vi "Initialize Master.vi"(8 "error in":errorcluster, 11 "Serial Master in":refnum<class "Serial Master.lvclass">) -> (0 "error out":errorcluster, 3 "Serial Master out":refnum<class "Serial Master.lvclass">)   [LabVIEW 2013, in "Modbus Library - Advance.lvlib" / "Serial Master.lvclass"]
doc: "This provides an interface for the master to open a connection to the slave."
uses:
  Serial Master.lvclass
  Serial Master.lvclass/Serial Master.ctl
  Transmission Data Unit/Serial Interface/Serial Data Unit.lvclass
  Read VISA resource name.vi
  Read Serial Data Unit.vi
  Read Baud Rate.vi
  Read Parity.vi
  Read Flow Control.vi
  Serial Shared Components/Serial Shared Components.lvlib
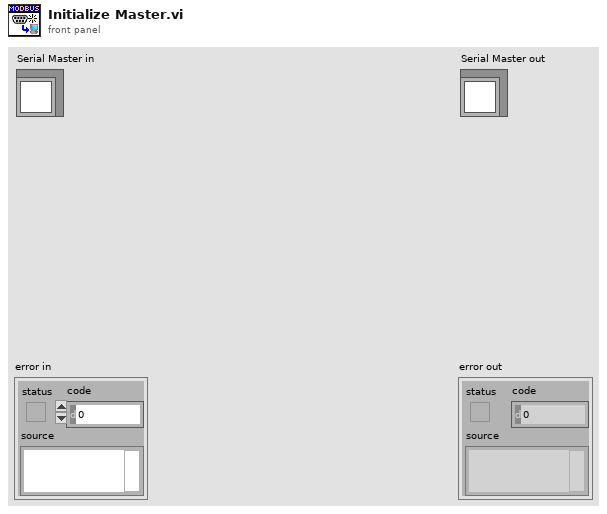
[diagram p1: front panel]
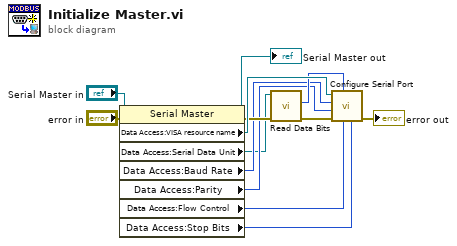
[diagram p0: block diagram]
diagram:
  n1 = property class="Serial Master"(reference="Serial Master in", error in="error in") -> (reference out=→"Serial Master out":refnum<class "Serial Master.lvclass">, error out=w11:errorcluster, "Data Access:VISA resource name"=w12:refnum<visa-resource-name>, "Data Access:Serial Data Unit"=w2:refnum<class "Serial Data Unit.lvclass">, "Data Access:Baud Rate"=w8:u32, "Data Access:Parity"=w7:u16, "Data Access:Flow Control"=w6:u16, "Data Access:Stop Bits"=w1:u16)
  n2 = call-dynamic "Read Data Bits.vi"("error in (no error)"=w11, "Serial Data Unit in"=w2) -> ("error out"=w10:errorcluster, "data bits"=w9:u16)  [unwired: 7 in, 1 out]
  n3 = call "Configure Serial Port.vi"("Stop Bits"=w1, "Flow Control"=w6, "data bits"=w9, "error in (no error)"=w10, "Parity"=w7, "Baud Rate"=w8, "VISA Refnum in"=w12) -> ("error out"=→"error out":errorcluster)  [unwired: 4 in]
